vi "ManualControlL0Sum.vi"() -> ()   [LabVIEW 2009]
uses:
  <vilib>/Utility/NIReport.llb/NI_report.lvclass
  <vilib>/Utility/NIReport.llb/HTML/NI_HTML.lvclass
panel:
  in  "Sum/Maj":bool
  in  "Ib Clip select":i32(slide) scale=0.0..63.0
  in  "Clipping Select":i32(slide) scale=1.0..3.0
  in  "Attenuation Select":i32(slide) scale=0.0..15.0
  in  "Delay Enable":i32(slide) scale=0.0..31.0
  in  "Channel Enable":i32(slide) scale=0.0..6.0
  in  "stop":bool
  in  "Instrument VISA in":T1={"AWG VISA"="generadorpulsos", "Oscilloscope  VISA "="Oscilloscope", "Integration Board IP"="172.16.7.43", "connection ID"=refnum, "report out"=refnum, "report file path"=path "C:/Documents and Settings/CTA_LAB01/Desktop/L0_Asic/L0 Asic Test Data"}
  out "error out":errorcluster
  in  "error in (no error)":errorcluster
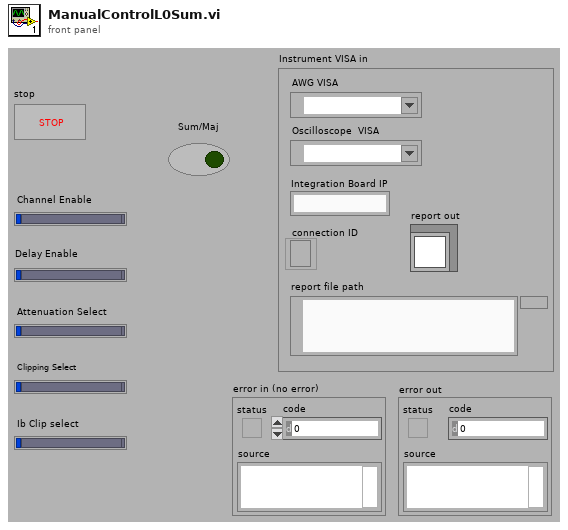
[diagram p1: front panel]
types:
  T1 = cluster{"AWG VISA":refnum<visa-resource-name>, "Oscilloscope  VISA ":refnum<visa-resource-name>, "Integration Board IP":string, "connection ID":refnum<k5>, "report out":refnum<class "NI_report.lvclass">, "report file path":path}
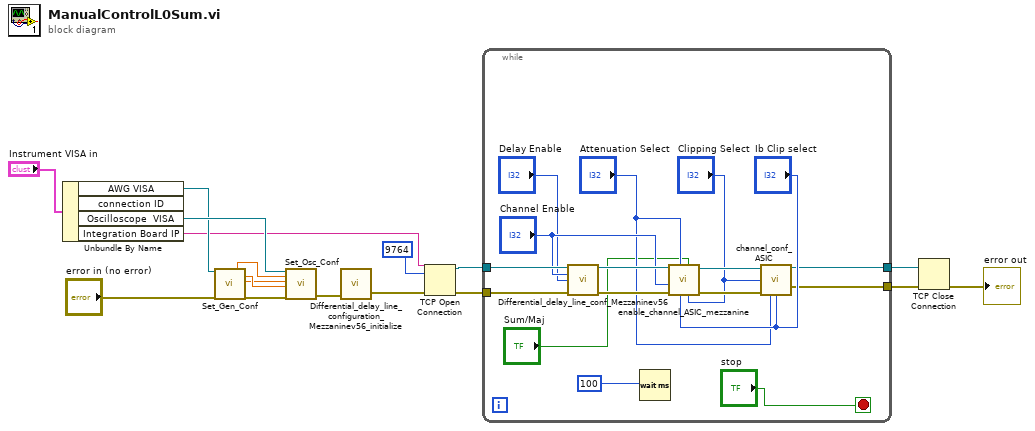
[diagram p0: block diagram]
diagram:
  n1 = Unbundle By Name("Instrument VISA in") -> ("AWG VISA"=w12:refnum<visa-resource-name>, "Oscilloscope  VISA"=w13:refnum<visa-resource-name>, "Integration Board IP"=w11:string)  [unwired: 1 out]
  n2 = call "Set_Gen_Conf.vi"("AWG VISA"=w12, "error in (no error)"="error in (no error)") -> ("Amplitude 1 OUT"=w9:dbl, "Pulse Width in seconds 1 OUT"=w8:dbl, "Trigger Level 1"=w7:dbl, "error out"=w15:errorcluster)  [unwired: 10 in, 4 out]
  n3 = call "Set_Osc_Conf.vi"("VISA resource name"=w13, "Amplitude IN"=w9, "Trigger Level IN"=w7, "Pulse Width in seconds IN"=w8, "error in (no error)"=w15) -> ("error out"=w6:errorcluster)  [unwired: 13 in, 1 out]
  n4 = call "Differential_delay_line_configuration_Mezzaninev56_initialize.vi"("error in (no error)"=w6) -> ("error out 2"=w5:errorcluster)  [unwired: 1 in]
  n5 = TCP Open Connection(address=w11, remote port or service name=9764, error in (no error)=w5) -> (connection ID=w2:refnum<k5>, error out=w4:errorcluster)  [unwired: 2 in]
  n6 = while {
    tunnel: w4 -> [w33]
    tunnel: [w18] -> w3
    tunnel: w2 -> [w30]
    tunnel: [w19] -> w1
    stop <- "stop" stop-if-true
    n7 = call "Differential_delay_line_conf_Mezzaninev56.vi"("connection ID"=w30, "channel"="Channel Enable", "Delay value"="Delay Enable", "error in (no error)"=w33) -> ("connection ID out"=w29:refnum<k5>, "error out 2"=w32:errorcluster)  [unwired: 4 in, 6 out]
    n8 = Wait (ms)(milliseconds to wait=100) -> ()  [unwired: 1 out]
    n9 = call "enable_channel_ASIC_mezzanine.vi"("Clip_sel_b"="Clipping Select", "maj/sum"="Sum/Maj", "Ib_clipVb"="Ib Clip select", "Att gain"="Attenuation Select", "error in"=w32, "Channel"="Channel Enable", "connection ID"=w29) -> ("error out"=w31:errorcluster, "connection ID out"=w28:refnum<k5>)  [unwired: 2 in, 1 out]
    n10 = call "channel_conf_ASIC.vi"("connection ID"=w28, "Clip_sel_b"="Clipping Select", "error out"=w31, "Att gain"="Attenuation Select", "Ib_ClipVb"="Ib Clip select") -> ("connection ID out"=w19:refnum<k5>, "error out 2"=w18:errorcluster)  [unwired: 6 in, 3 out]
  }
  n11 = TCP Close Connection(connection ID=w1, error in (no error)=w3) -> (error out=→"error out":errorcluster)  [unwired: 1 in, 1 out]
